vi "Write to File Serial Numbers.vi"(8 "error in":errorcluster, 10 "Serial Numbers Array":string[](array[string]), 11 "Refnum in":T1) -> (0 "error out":errorcluster, 3 "refnum out":T1)   [LabVIEW 2018]
uses:
  <vilib>/Utility/config.llb/Config Data RefNum.ctl
  <vilib>/Utility/config.llb/Write Key (String).vi
  <vilib>/Utility/config.llb/NI_LVConfig.lvlib
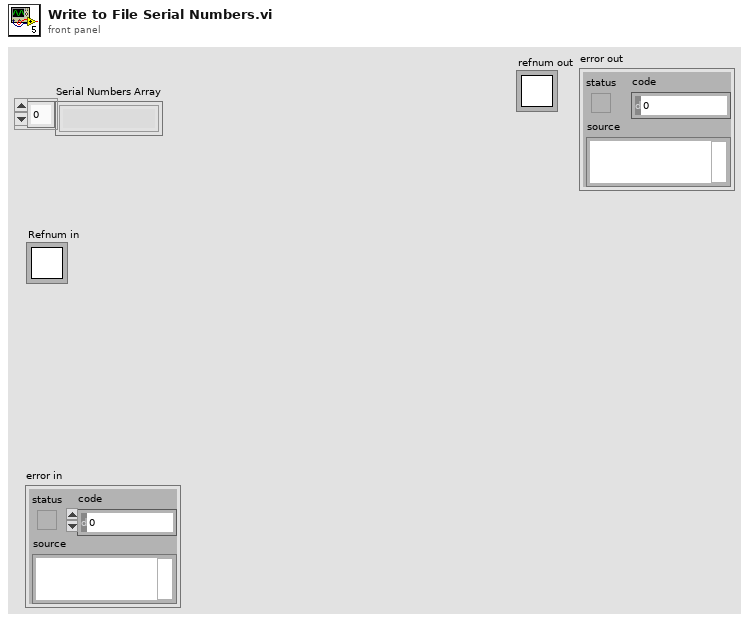
[diagram p1: front panel]
types:
  T1 = typedef "NI_LVConfig.lvlib/Config Data RefNum.ctl" = refnum<k1>
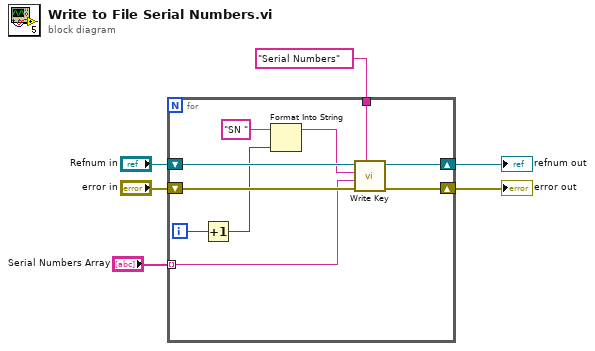
[diagram p0: block diagram]
diagram:
  n1 = for {
    shift-right: [w10] -> w4
    shift-left: "Refnum in" -> [w16]
    shift-right: [w9] -> w3
    shift-left: "error in" -> [w15]
    tunnel: "Serial Numbers" ("Shift") -> [w14]
    tunnel: "Serial Numbers Array" -> [w7] mode=indexing
    i -> [w11]
    n2 = Increment(x=w11) -> (x+1=w8:i32)
    n3 = Format Into String(initial string="SN " ("key"), w8) -> (resulting string=w12:string)  [unwired: 2 in, 1 out]
    n4 = call-poly <vilib>:"Write Key.vi"("section"=w14, "error in (no error)"=w15, "value"=w7, "key"=w12, "refnum"=w16) -> ("error out"=w9:errorcluster, "refnum out"=w10:T1)  [unwired: 4 in, 1 out]
  }
  "refnum out" <- w4
  "error out" <- w3
